vi "Configuration Parse.vi"(8 "error in":errorcluster, 11 "UI Controls":T5={"measurement configuration"={"Automation Test"=FALSE, "Power sequencing file path"="", "SMU name"="", "SMU channel"="0", "RFSG name"="", "RFSG port"="", "RFSG attenuation mode"=enum."<None>", "RFSG external attenuation (dB)"=0.0, "RFSG s-parameters orientation"=enum."Port1 Towards DUT", "RFSG s2p file path"="", "RFmx name"="", "RFmx port"="", "RFmx attenuation mode"=enum."<None>", "RFmx external attenuation (dB)"=0.0, "RFmx attenuation path name"="", "RFmx s-parameters orientation"=enum."Port1 Towards DUT", "RFmx attenuation s2p path name"="", "RFmx s2p file path"="", "Compression_Expected DUT Gain (dB)"=0.0, "Compression_Max Linear Range (dBm)"=0.0, "Compression_Compression Point (dB)"=0.0, "Compression_Target Pin (dBm)"=1.0, "Compression_RFSG Frequency Start (Hz)"=0.0, "Compression_RFSG Frequency Stop (Hz)"=0.0, "Compression_RFSG Number of Frequency Step"=0, "Compression_RFSG Power Start (dBm)"=0.0, "Compression_RFSG Power Stop(dBm)"=0.0, "Compression_RFSG Power Step Size (dB)"=0.0, "Compression_RBW (Hz)"=0.0, "Compression_RF Measurement Interval (s)"=0.0, "Compression_DC Measurement Interval (s)"=0.001, "Compression_Stimulus Mode"=enum."Constant Power and RF", "CP_CW_DC Source Delay (s)"=0.0, "CP_PRF_DC Source Delay (s)"=0.0, "CP_PRF_RFmx Trigger Delay (s)"=0.0, "CP_PRF_RF Pulse Width (s)"=0.0001, "CP_PRF_PRI (s)"=0.001, "PP_PRF_DC Source Delay (s)"=0.0, "PP_PRF_RFmx Trigger Delay (s)"=0.0, "PP_PRF_RF Pulse Width (s)"=0.0001, "PP_PRF_PRI (s)"=0.001, "PP_PRF_DC Pulse Width (s)"=0.0008, "PP_PRF_ON Current Limit (A)"=2.0, "PP_PRF_Bias Voltage Level (V)"=0.0, "PP_PRF_Bias Current Limit (A)"=0.2}, "measurement results"={"Status"="", "per Freq Plot Names"=[], "Linear Gain vs Freq"=[], "OPxdB vs Freq"=[], "Pout@Pin vs Freq"=[], "Gain@Pin vs Freq"=[], "PAE@Pin vs Freq"=[], "Pout vs Pin per Freq"=[], "Gain vs Pin per Freq"=[], "PAE vs Pin per Freq"=[], "Pout@Pin (Mean)"=0.0, "Gain@Pin (Mean)"=0.0, "PAE@Pin (Mean)"=0.0, "Linear Gain (Mean)"=0.0, "OPxdB (Mean)"=0.0}} {"measurement configuration"."Compression_Target Pin (dBm)" format="%#pdBm"; "measurement configuration"."PP_PRF_Bias Current Limit (A)" format="%#pA"; "measurement configuration"."PP_PRF_Bias Voltage Level (V)" format="%#pV"; "measurement configuration"."PP_PRF_ON Current Limit (A)" format="%#pA"; "measurement configuration"."PP_PRF_DC Pulse Width (s)" format="%#ps"; "measurement configuration"."PP_PRF_PRI (s)" format="%#ps"; "measurement configuration"."PP_PRF_RF Pulse Width (s)" format="%#ps"; "measurement configuration"."PP_PRF_RFmx Trigger Delay (s)" format="%#ps"; "measurement configuration"."PP_PRF_DC Source Delay (s)" format="%#ps"; "measurement configuration"."CP_PRF_PRI (s)" format="%#ps"; "measurement configuration"."CP_PRF_RF Pulse Width (s)" format="%#ps"; "measurement configuration"."CP_PRF_RFmx Trigger Delay (s)" format="%#ps"; "measurement configuration"."CP_PRF_DC Source Delay (s)" format="%#ps"; "measurement configuration"."CP_CW_DC Source Delay (s)" format="%#ps"; "measurement configuration"."Compression_DC Measurement Interval (s)" format="%#ps"; "measurement configuration"."Compression_RF Measurement Interval (s)" format="%#ps"; "measurement configuration"."RFmx external attenuation (dB)" format="%.2f"; "measurement configuration"."RFSG external attenuation (dB)" format="%.2f"}) -> (0 "error out":errorcluster, 1 "RFmx Settings":T7 {"Attenuation"."s2p File"."RFmx S-Parameters Orientation" items=["Port1 Towards DUT"=24000, "Port2 Towards DUT"=24001]; "Attenuation"."Constant Attenuation"."RFmx External Attenuation (dB)" format="%.2f"}, 2 "RFSG Settings":T6 {"Attenuation"."s2p File"."RFSG S-parameters Orientation" items=["Port1 Towards DUT"=24000, "Port2 Towards DUT"=24001]; "Attenuation"."Contant Attenuation"."RFSG External Attenuation (dB)" format="%.2f"}, 3 "Test Configuration":T2={"Expected DUT Gain (dB)"=0.0, "Max Linear Range (dBm)"=0.0, "Compression Point (dB)"=0.0, "Pout at Pin (dBm)"=1.0, "RFSG Frequency Start (Hz)"=0.0, "RFSG Frequency Stop (Hz)"=0.0, "RFSG Number of Frequency Step"=0, "Power Start (dBm)"=0.0, "Power Stop(dBm)"=0.0, "Power Step Size (dB)"=0.0, "RBW (Hz)"=0.0, "Modes"={"RF Measurement Interval (s)"=0.001, "DC Measurement Interval (s)"=0.0, "Power Stimulus Mode"=enum."Constant Power and RF", "CP_CW_DC Source Delay (s)"=0.0002, "CP_PRF_RF Pulse Width (s)"=0.0009, "CP_PRF_PRI (s)"=0.015, "CP_PRF_DC Source Delay (s)"=0.0, "CP_PRF_RFmx Trigger Delay (s)"=0.2, "PP_PRF_RF Pulse Width (s)"=0.0, "PP_PRF_PRI (s)"=0.0, "PP_PRF_DC Pulse Width (s)"=0.0008, "PP_PRF_Bias Voltage Level (V)"=0.0, "PP_PRF_Bias Current Limit (A)"=0.2, "PP_PRF_DC Source Delay (s)"=0.0, "PP_PRF_RFmx Trigger Delay (s)"=0.0}} {"Pout at Pin (dBm)" format="%#pdBm"; "Modes"."PP_PRF_RFmx Trigger Delay (s)" format="%#ps"; "Modes"."PP_PRF_DC Source Delay (s)" format="%#ps"; "Modes"."PP_PRF_Bias Current Limit (A)" format="%#pA"; "Modes"."PP_PRF_Bias Voltage Level (V)" format="%#pV"; "Modes"."PP_PRF_DC Pulse Width (s)" format="%#ps"; "Modes"."PP_PRF_PRI (s)" format="%#ps"; "Modes"."PP_PRF_RF Pulse Width (s)" format="%#ps"; "Modes"."CP_PRF_RFmx Trigger Delay (s)" format="%#ps"; "Modes"."CP_PRF_DC Source Delay (s)" format="%#ps"; "Modes"."CP_PRF_PRI (s)" format="%#ps"; "Modes"."CP_PRF_RF Pulse Width (s)" format="%#ps"; "Modes"."CP_CW_DC Source Delay (s)" format="%#ps"; "Modes"."DC Measurement Interval (s)" format="%#_6p"; "RFSG Frequency Stop (Hz)" format="%#_6p"; "Power Start (dBm)" format="%#_6p"; "Power Stop(dBm)" format="%#_6p"; "RFSG Frequency Start (Hz)" format="%#_6p"; "Expected DUT Gain (dB)" step=1.0 format="%#_6p"}, 5 "SMU Settings":T1={"SMU Name"="PXI1Slot15", "SMU Channel"="2", "IDD Current Limit (A)"=0.0})   [LabVIEW 2023, in "FPT_Compression.lvclass"]
uses:
  FPT_Compression.lvclass
  Measurement/Controls/RFmx Config - Compression.ctl
  Measurement/Controls/RFSG Config - Compression.ctl
  Measurement Configuration.ctl
  Measurement Results.ctl
  Measurement/Controls/Test Config - Compression.ctl
  Measurement/Controls/SMU Config - Compression.ctl
  FPT_Compression.lvclass/FPT_Compression.ctl
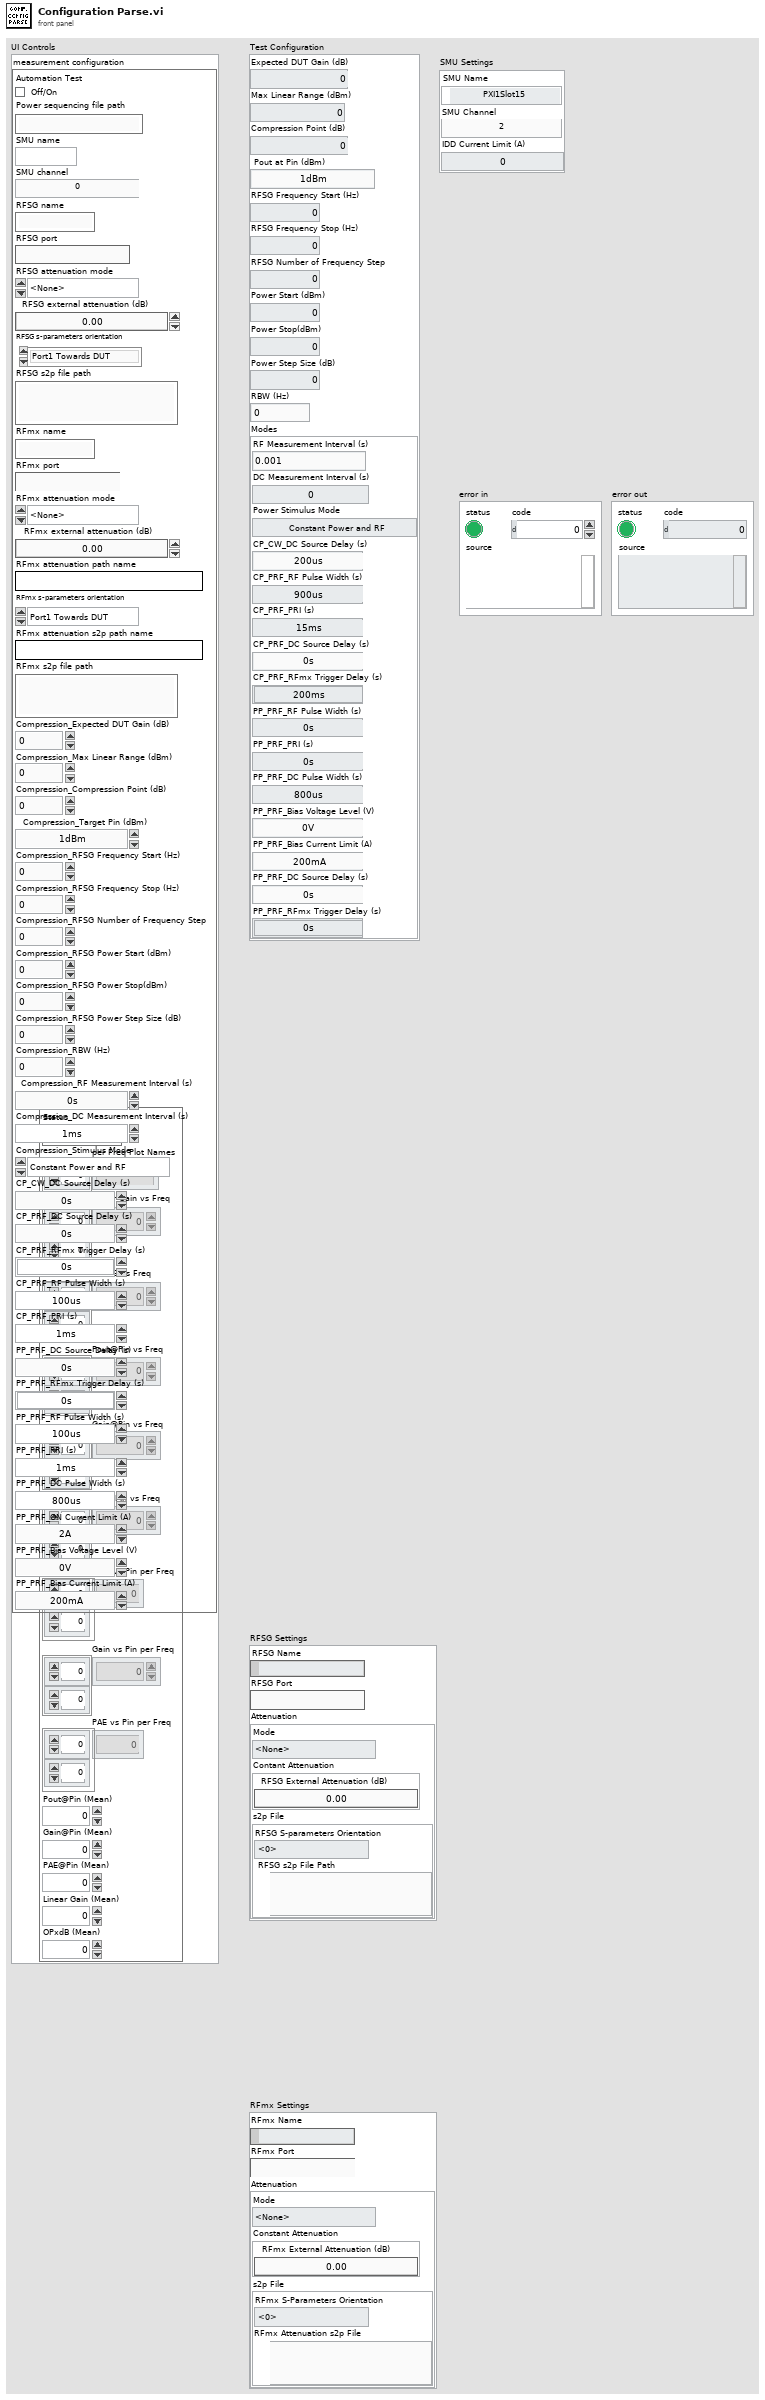
[diagram p1: front panel]
types:
  T1 = typedef "SMU Config - Compression.ctl" = cluster{"SMU Name":refnum<k15>, "SMU Channel":string, "IDD Current Limit (A)":dbl}
  T2 = typedef "Test Config - Compression.ctl" = cluster{"Expected DUT Gain (dB)":dbl, "Max Linear Range (dBm)":dbl, "Compression Point (dB)":dbl, "Pout at Pin (dBm)":dbl, "RFSG Frequency Start (Hz)":dbl, "RFSG Frequency Stop (Hz)":dbl, "RFSG Number of Frequency Step":i32, "Power Start (dBm)":dbl, "Power Stop(dBm)":dbl, "Power Step Size (dB)":dbl, "RBW (Hz)":dbl, "Modes":cluster{"RF Measurement Interval (s)":dbl, "DC Measurement Interval (s)":dbl, "Power Stimulus Mode":enum16{"Constant Power and RF", "Constant Power and Pulsed RF", "Pulsed Power and RF"}, "CP_CW_DC Source Delay (s)":dbl, "CP_PRF_RF Pulse Width (s)":dbl, "CP_PRF_PRI (s)":dbl, "CP_PRF_DC Source Delay (s)":dbl, "CP_PRF_RFmx Trigger Delay (s)":dbl, "PP_PRF_RF Pulse Width (s)":dbl, "PP_PRF_PRI (s)":dbl, "PP_PRF_DC Pulse Width (s)":dbl, "PP_PRF_Bias Voltage Level (V)":dbl, "PP_PRF_Bias Current Limit (A)":dbl, "PP_PRF_DC Source Delay (s)":dbl, "PP_PRF_RFmx Trigger Delay (s)":dbl}}
  T3 = typedef "FPT_Compression.lvclass/Measurement Configuration.ctl" = cluster{"Automation Test":bool, "Power sequencing file path":string, "SMU name":string, "SMU channel":string, "RFSG name":string, "RFSG port":string, "RFSG attenuation mode":enum32{"<None>", "Constant Attenuation", "s2p File"}, "RFSG external attenuation (dB)":dbl, "RFSG s-parameters orientation":enum32{"Port1 Towards DUT", "Port2 Towards DUT"}, "RFSG s2p file path":string, "RFmx name":string, "RFmx port":string, "RFmx attenuation mode":enum32{"<None>", "Constant Attenuation", "s2p File"}, "RFmx external attenuation (dB)":dbl, "RFmx attenuation path name":string, "RFmx s-parameters orientation":enum32{"Port1 Towards DUT", "Port2 Towards DUT"}, "RFmx attenuation s2p path name":string, "RFmx s2p file path":string, "Compression_Expected DUT Gain (dB)":dbl, "Compression_Max Linear Range (dBm)":dbl, "Compression_Compression Point (dB)":dbl, "Compression_Target Pin (dBm)":dbl, "Compression_RFSG Frequency Start (Hz)":dbl, "Compression_RFSG Frequency Stop (Hz)":dbl, "Compression_RFSG Number of Frequency Step":i32, "Compression_RFSG Power Start (dBm)":dbl, "Compression_RFSG Power Stop(dBm)":dbl, "Compression_RFSG Power Step Size (dB)":dbl, "Compression_RBW (Hz)":dbl, "Compression_RF Measurement Interval (s)":dbl, "Compression_DC Measurement Interval (s)":dbl, "Compression_Stimulus Mode":enum32{"Constant Power and RF", "Constant Power and Pulsed RF", "Pulsed Power and RF"}, "CP_CW_DC Source Delay (s)":dbl, "CP_PRF_DC Source Delay (s)":dbl, "CP_PRF_RFmx Trigger Delay (s)":dbl, "CP_PRF_RF Pulse Width (s)":dbl, "CP_PRF_PRI (s)":dbl, "PP_PRF_DC Source Delay (s)":dbl, "PP_PRF_RFmx Trigger Delay (s)":dbl, "PP_PRF_RF Pulse Width (s)":dbl, "PP_PRF_PRI (s)":dbl, "PP_PRF_DC Pulse Width (s)":dbl, "PP_PRF_ON Current Limit (A)":dbl, "PP_PRF_Bias Voltage Level (V)":dbl, "PP_PRF_Bias Current Limit (A)":dbl}
  T4 = typedef "FPT_Compression.lvclass/Measurement Results.ctl" = cluster{"Status":string, "per Freq Plot Names":string[], "Linear Gain vs Freq":dbl[][], "OPxdB vs Freq":dbl[][], "Pout@Pin vs Freq":dbl[][], "Gain@Pin vs Freq":dbl[][], "PAE@Pin vs Freq":dbl[][], "Pout vs Pin per Freq":dbl[][], "Gain vs Pin per Freq":dbl[][], "PAE vs Pin per Freq":dbl[][], "Pout@Pin (Mean)":dbl, "Gain@Pin (Mean)":dbl, "PAE@Pin (Mean)":dbl, "Linear Gain (Mean)":dbl, "OPxdB (Mean)":dbl}
  T5 = cluster{"measurement configuration":T3, "measurement results":T4}
  T6 = typedef "RFSG Config - Compression.ctl" = cluster{"RFSG Name":refnum<k15>, "RFSG Port":string, "Attenuation":cluster{"Mode":enum32{"<None>", "Constant Attenuation", "s2p File"}, "Contant Attenuation":cluster{"RFSG External Attenuation (dB)":dbl}, "s2p File":cluster{"RFSG S-parameters Orientation":i32, "RFSG s2p File Path":path}}}
  T7 = typedef "RFmx Config - Compression.ctl" = cluster{"RFmx Name":refnum<k15>, "RFmx Port":string, "Attenuation":cluster{"Mode":enum32{"<None>", "Constant Attenuation", "s2p File"}, "Constant Attenuation":cluster{"RFmx External Attenuation (dB)":dbl}, "s2p File":cluster{"RFmx S-Parameters Orientation":i32, "RFmx Attenuation s2p File":path}}}
  T8 = enum32{"<None>", "Constant Attenuation", "s2p File"}
  T9 = enum32{"Constant Power and RF", "Constant Power and Pulsed RF", "Pulsed Power and RF"}
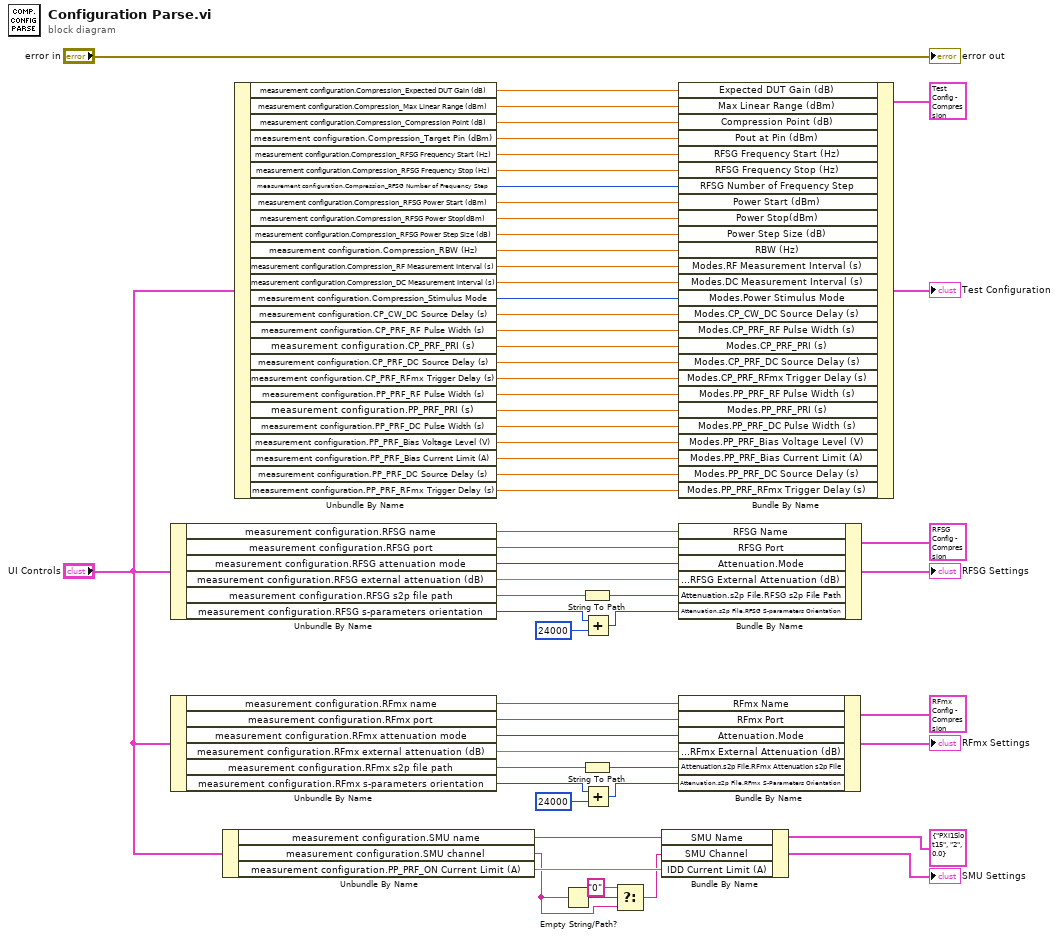
[diagram p0: block diagram]
diagram:
  n1 = Unbundle By Name("UI Controls") -> ("measurement configuration.RFSG name"=w38:string, "measurement configuration.RFSG port"=w47:string, "measurement configuration.RFSG attenuation mode"=w32:T8, "measurement configuration.RFSG external attenuation (dB)"=w39:dbl, "measurement configuration.RFSG s2p file path"=w43:string, "measurement configuration.RFSG s-parameters orientation"=w31:enum32{"Port1 Towards DUT", "Port2 Towards DUT"})
  n2 = Unbundle By Name("UI Controls") -> ("measurement configuration.RFmx name"=w41:string, "measurement configuration.RFmx port"=w48:string, "measurement configuration.RFmx attenuation mode"=w33:T8, "measurement configuration.RFmx external attenuation (dB)"=w42:dbl, "measurement configuration.RFmx s2p file path"=w46:string, "measurement configuration.RFmx s-parameters orientation"=w27:enum32{"Port1 Towards DUT", "Port2 Towards DUT"})
  n3 = Unbundle By Name("UI Controls") -> ("measurement configuration.SMU name"=w7:string, "measurement configuration.SMU channel"=w2:string, "measurement configuration.PP_PRF_ON Current Limit (A)"=w6:dbl)
  n4 = Unbundle By Name("UI Controls") -> ("measurement configuration.Compression_Expected DUT Gain (dB)"=w49:dbl, "measurement configuration.Compression_Max Linear Range (dBm)"=w50:dbl, "measurement configuration.Compression_Compression Point (dB)"=w51:dbl, "measurement configuration.Compression_Target Pin (dBm)"=w5:dbl, "measurement configuration.Compression_RFSG Frequency Start (Hz)"=w52:dbl, "measurement configuration.Compression_RFSG Frequency Stop (Hz)"=w53:dbl, "measurement configuration.Compression_RFSG Number of Frequency Step"=w54:i32, "measurement configuration.Compression_RFSG Power Start (dBm)"=w55:dbl, "measurement configuration.Compression_RFSG Power Stop(dBm)"=w56:dbl, "measurement configuration.Compression_RFSG Power Step Size (dB)"=w57:dbl, "measurement configuration.Compression_RBW (Hz)"=w58:dbl, "measurement configuration.Compression_RF Measurement Interval (s)"=w25:dbl, "measurement configuration.Compression_DC Measurement Interval (s)"=w24:dbl, "measurement configuration.Compression_Stimulus Mode"=w23:T9, "measurement configuration.CP_CW_DC Source Delay (s)"=w22:dbl, "measurement configuration.CP_PRF_RF Pulse Width (s)"=w21:dbl, "measurement configuration.CP_PRF_PRI (s)"=w20:dbl, "measurement configuration.CP_PRF_DC Source Delay (s)"=w19:dbl, "measurement configuration.CP_PRF_RFmx Trigger Delay (s)"=w18:dbl, "measurement configuration.PP_PRF_RF Pulse Width (s)"=w17:dbl, "measurement configuration.PP_PRF_PRI (s)"=w16:dbl, "measurement configuration.PP_PRF_DC Pulse Width (s)"=w15:dbl, "measurement configuration.PP_PRF_Bias Voltage Level (V)"=w14:dbl, "measurement configuration.PP_PRF_Bias Current Limit (A)"=w13:dbl, "measurement configuration.PP_PRF_DC Source Delay (s)"=w12:dbl, "measurement configuration.PP_PRF_RFmx Trigger Delay (s)"=w11:dbl)
  n5 = Empty String/Path?(string/path=w2) -> (empty?=w4:bool)
  n6 = String To Path(string=w43) -> (path=w44:path)
  n7 = String To Path(string=w46) -> (path=w45:path)
  n8 = Add(x=w31, y=u32 24000) -> (x+y=w29:u32)
  n9 = Add(x=w27, y=u32 24000) -> (x+y=w26:u32)
  n10 = Select(t="0", s=w4, f=w2) -> (s? t:f=w3:string)
  n11 = Bundle By Name(cluster=T1 {"SMU Name"="PXI1Slot15", "SMU Channel"="2", "IDD Current Limit (A)"=0.0} ("SMU Settings"), "SMU Name"=w7, "SMU Channel"=w3, "IDD Current Limit (A)"=w6) -> (→"SMU Settings":T1)
  n12 = Bundle By Name(cluster=T2 {"Expected DUT Gain (dB)"=0.0, "Max Linear Range (dBm)"=0.0, "Compression Point (dB)"=0.0, "Pout at Pin (dBm)"=1.0, "RFSG Frequency Start (Hz)"=0.0, "RFSG Frequency Stop (Hz)"=0.0, "RFSG Number of Frequency Step"=0, "Power Start (dBm)"=0.0, "Power Stop(dBm)"=0.0, "Power Step Size (dB)"=0.0, "RBW (Hz)"=0.0, "Modes"={"RF Measurement Interval (s)"=0.001, "DC Measurement Interval (s)"=0.0, "Power Stimulus Mode"=enum."Constant Power and RF", "CP_CW_DC Source Delay (s)"=0.0002, "CP_PRF_RF Pulse Width (s)"=0.0009, "CP_PRF_PRI (s)"=0.015, "CP_PRF_DC Source Delay (s)"=0.0, "CP_PRF_RFmx Trigger Delay (s)"=0.2, "PP_PRF_RF Pulse Width (s)"=0.0, "PP_PRF_PRI (s)"=0.0, "PP_PRF_DC Pulse Width (s)"=0.0008, "PP_PRF_Bias Voltage Level (V)"=0.0, "PP_PRF_Bias Current Limit (A)"=0.2, "PP_PRF_DC Source Delay (s)"=0.0, "PP_PRF_RFmx Trigger Delay (s)"=0.0}} ("Test Configuration"), "Expected DUT Gain (dB)"=w49, "Max Linear Range (dBm)"=w50, "Compression Point (dB)"=w51, "Pout at Pin (dBm)"=w5, "RFSG Frequency Start (Hz)"=w52, "RFSG Frequency Stop (Hz)"=w53, "RFSG Number of Frequency Step"=w54, "Power Start (dBm)"=w55, "Power Stop(dBm)"=w56, "Power Step Size (dB)"=w57, "RBW (Hz)"=w58, "Modes.RF Measurement Interval (s)"=w25, "Modes.DC Measurement Interval (s)"=w24, "Modes.Power Stimulus Mode"=w23, "Modes.CP_CW_DC Source Delay (s)"=w22, "Modes.CP_PRF_RF Pulse Width (s)"=w21, "Modes.CP_PRF_PRI (s)"=w20, "Modes.CP_PRF_DC Source Delay (s)"=w19, "Modes.CP_PRF_RFmx Trigger Delay (s)"=w18, "Modes.PP_PRF_RF Pulse Width (s)"=w17, "Modes.PP_PRF_PRI (s)"=w16, "Modes.PP_PRF_DC Pulse Width (s)"=w15, "Modes.PP_PRF_Bias Voltage Level (V)"=w14, "Modes.PP_PRF_Bias Current Limit (A)"=w13, "Modes.PP_PRF_DC Source Delay (s)"=w12, "Modes.PP_PRF_RFmx Trigger Delay (s)"=w11) -> (→"Test Configuration":T2)
  n13 = Bundle By Name(cluster=T6 {"RFSG Name"="5842_0", "RFSG Port"="", "Attenuation"={"Mode"=enum."Constant Attenuation", "Contant Attenuation"={"RFSG External Attenuation (dB)"=2.0}, "s2p File"={"RFSG S-parameters Orientation"=24000, "RFSG s2p File Path"=path ""}}} ("RFSG Settings"), "RFSG Name"=w38, "RFSG Port"=w47, "Attenuation.Mode"=w32, "Attenuation.Contant Attenuation.RFSG External Attenuation (dB)"=w39, "Attenuation.s2p File.RFSG s2p File Path"=w44, "Attenuation.s2p File.RFSG S-parameters Orientation"=w29) -> (→"RFSG Settings":T6)
  n14 = Bundle By Name(cluster=T7 {"RFmx Name"="5842_0", "RFmx Port"="", "Attenuation"={"Mode"=enum."Constant Attenuation", "Constant Attenuation"={"RFmx External Attenuation (dB)"=1.2}, "s2p File"={"RFmx S-Parameters Orientation"=24000, "RFmx Attenuation s2p File"=path ""}}} ("RFmx Settings"), "RFmx Name"=w41, "RFmx Port"=w48, "Attenuation.Mode"=w33, "Attenuation.Constant Attenuation.RFmx External Attenuation (dB)"=w42, "Attenuation.s2p File.RFmx Attenuation s2p File"=w45, "Attenuation.s2p File.RFmx S-Parameters Orientation"=w26) -> (→"RFmx Settings":T7)
  "error out" <- "error in"
